vi "Convert String to NT String Buffer.vi"(11 "LV Buffer":string) -> (3 "NT Buffer":string)   [LabVIEW 2017]
doc: "Pack the LV string so that it conforms to the Java and C++ client format. It changes the length to LEB128 encoding."
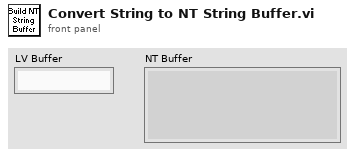
[diagram p1: front panel]
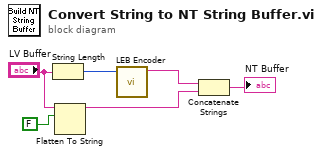
[diagram p0: block diagram]
diagram:
  n1 = String Length(string="LV Buffer") -> (length=w2:i32)
  n2 = Flatten To String(anything="LV Buffer", prepend array or string size? (T)=FALSE) -> (data string=w4:string)  [unwired: 2 in, 2 out]
  n3 = call <vilib>:"LEB Encoder.vi"("Number"=w2) -> ("encoded string"=w1:string)  [unwired: 10 in]
  n4 = Concatenate Strings(w1, w4) -> (→"NT Buffer":string)
